vi "Rotate Int String Number (SubVI).vi"(11 "Int Number In":i32 format="%08x") -> (1 "Rotated Int String":string, 2 "*(type *) &x":i32, 3 "Orig String":string)   [LabVIEW 2017, in "LV_Unicorn.lvlib"]
uses:
  LV_Unicorn.lvlib
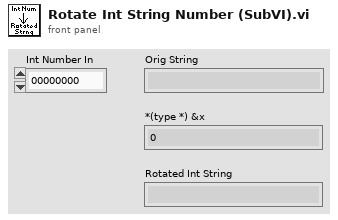
[diagram p1: front panel]
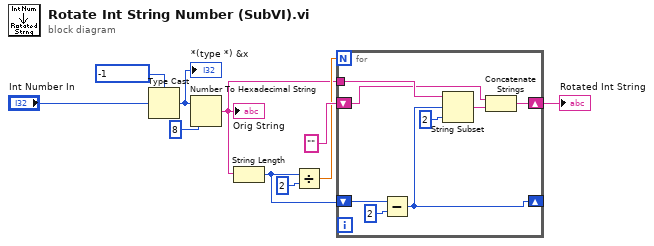
[diagram p0: block diagram]
diagram:
  n1 = Type Cast(type=-1, x="Int Number In") -> (*(type *) &x=w4:i32)
  "*(type *) &x" <- w4
  n2 = Number To Hexadecimal String(1:i16 8 ("width (-)"), 2:w4) -> (0:w5:string)
  "Orig String" <- w5
  n3 = String Length(string=w5) -> (length=w8:i32)
  n4 = Divide(x=w8, y=2) -> (x/y=w6:dbl)
  n5 = for {
    N: w6 -> [_]
    tunnel: w5 -> [w18]
    shift-right: [w11] -> _
    shift-left: w8 -> [w17]
    shift-right: [w12] -> w10
    shift-left: "" -> [w14]
    n6 = Subtract(x=w17, y=2) -> (x-y=w11:i32)
    n7 = String Subset(string=w18, offset (0)=w11, length (rest)=2 ("length (rest)")) -> (substring=w13:string)
    n8 = Concatenate Strings(w14, w13) -> (w12:string)
  }
  "Rotated Int String" <- w10
